vi "Solve2.vi"(8 "Error In":errorcluster, 11 "object in":refnum<class "2021_4.lvclass">) -> (0 "Error Out":errorcluster, 2 "Result":u64, 3 "object out":refnum<class "2021_4.lvclass">)   [LabVIEW 2020, in "2021_4.lvclass"]
uses:
  2021_4.lvclass
  2021_4.lvclass/2021_4.ctl
panel:
  out "LastBoard":i32
  out "Boards":bool[][][](array[boolean])
  out "Board":i32
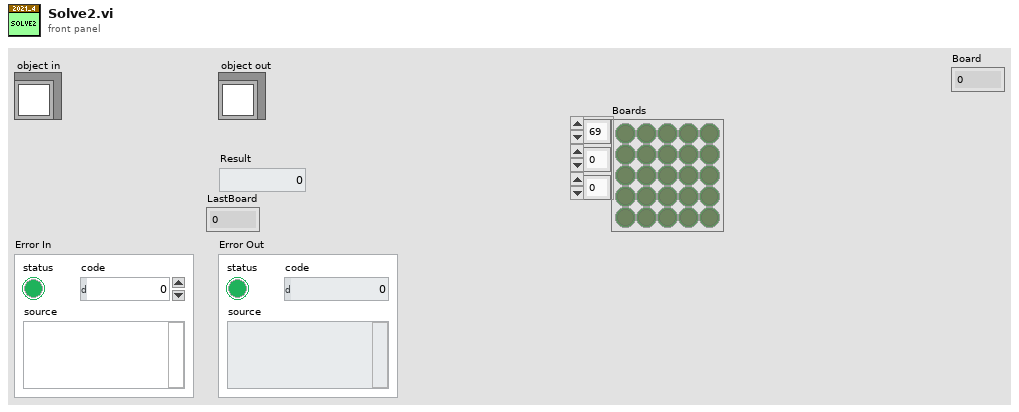
[diagram p1: front panel]
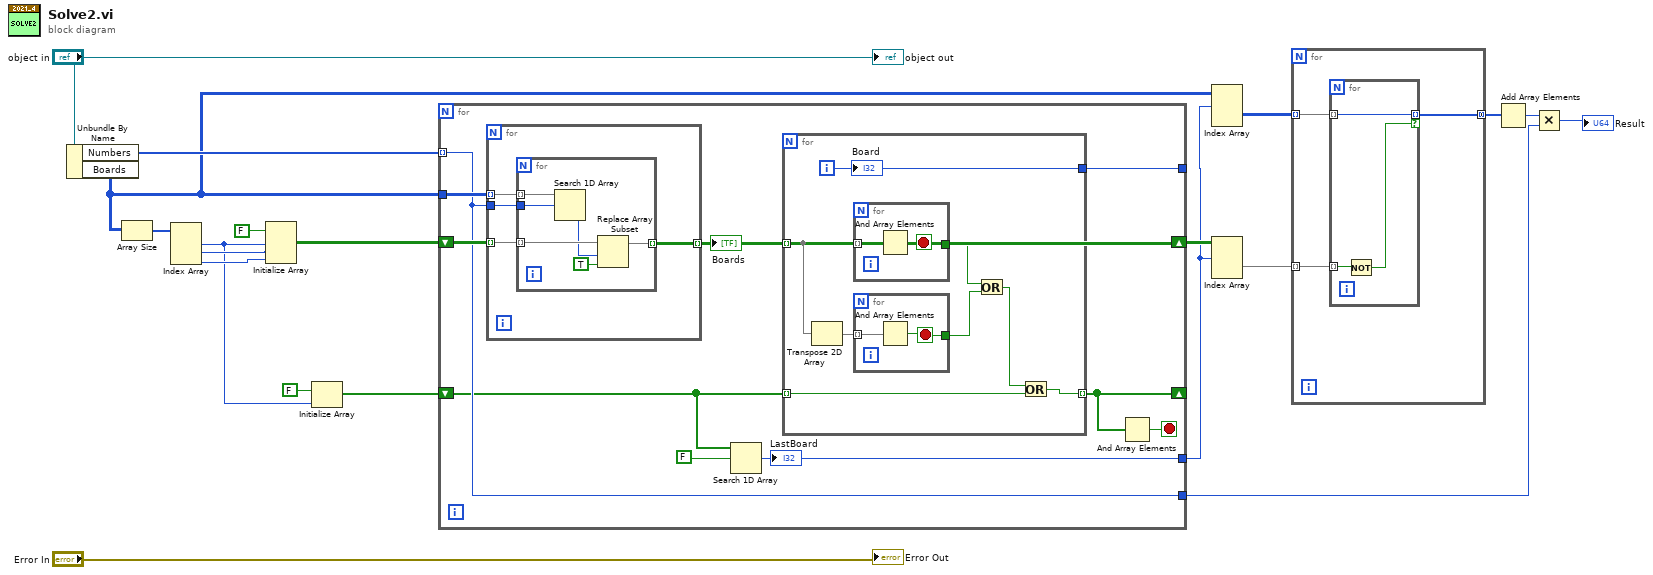
[diagram p0: block diagram]
diagram:
  n1 = Unbundle By Name("object in") -> ("Numbers"=w14:u32[], "Boards"=w12:i32[][][])
  n2 = Array Size(array=w12) -> (size(s)=w18:i32[])
  n3 = Index Array(array=w18) -> (element #1=w4:i32, element #2=w17:i32, element #3=w16:i32)  [unwired: 3 in]
  n4 = Initialize Array(FALSE, w4, w17, w16) -> (w13:bool[][][])
  n5 = Initialize Array(FALSE, w4) -> (w2:bool[])
  n6 = for {
    tunnel: w14 -> [w26] mode=indexing
    tunnel: w12 -> [w29]
    shift-right: [w28] -> w10
    shift-left: w13 -> [w30]
    tunnel: [w27] -> _
    tunnel: [w26] -> w6
    shift-right: [w25] -> _
    shift-left: w2 -> [w23]
    tunnel: [w21] -> w1
    stop <- w24 stop-if-true
    n7 = for {
      tunnel: w30 -> [w45] mode=indexing
      tunnel: w29 -> [w46] mode=indexing
      tunnel: w26 -> [w44]
      tunnel: [w43] -> w28 mode=indexing
      n8 = for {
        tunnel: w46 -> [w52] mode=indexing
        tunnel: w45 -> [w50] mode=indexing
        tunnel: w44 -> [w51]
        tunnel: [w47] -> w43 mode=indexing
        n9 = Search 1D Array(1D array=w52, element=w51) -> (index of element=w49:i32)  [unwired: 1 in]
        n10 = Replace Array Subset(array=w50, new element=TRUE ("new element/subarray"), index=w49) -> (w47:bool[])
      }
    }
    "Boards" <- w28
    n11 = Search 1D Array(1D array=w23, element=FALSE) -> (index of element=w21:i32)  [unwired: 1 in]
    "LastBoard" <- w21
    n12 = for {
      tunnel: w28 -> [w38] mode=indexing
      tunnel: [w34] -> w27
      tunnel: w23 -> [w33] mode=indexing
      tunnel: [w31] -> w25 mode=indexing
      i -> [w34]
      n13 = Transpose 2D Array(2D array=w38) -> (transposed array=w37:bool[][])
      n14 = for {
        tunnel: w38 -> [w42] mode=indexing
        tunnel: [w41] -> w36
        stop <- w41 stop-if-true
        n15 = And Array Elements(Boolean array=w42) -> (logical AND=w41:bool)
      }
      n16 = for {
        tunnel: w37 -> [w40] mode=indexing
        tunnel: [w39] -> w35
        stop <- w39 stop-if-true
        n17 = And Array Elements(Boolean array=w40) -> (logical AND=w39:bool)
      }
      n18 = Or(x=w36, y=w35) -> (x .or. y?=w32:bool)
      n19 = Or(x=w32, y=w33) -> (x .or. y?=w31:bool)
      "Board" <- w34
    }
    n20 = And Array Elements(Boolean array=w25) -> (logical AND=w24:bool)
  }
  n21 = Index Array(array=w12, index (dim 0)=w1) -> (element=w11:i32[][])  [unwired: 2 in]
  n22 = Index Array(array=w10, index (dim 0)=w1) -> (element=w9:bool[][])  [unwired: 2 in]
  n23 = for {
    tunnel: w11 -> [w55] mode=indexing
    tunnel: w9 -> [w54] mode=indexing
    tunnel: [w53] -> w8 mode=concatenating
    n24 = for {
      tunnel: w55 -> [w58] mode=indexing
      tunnel: w54 -> [w57] mode=indexing
      tunnel: [w58] -> w53 mode=indexing if=w56
      n25 = Not(x=w57) -> (.not. x?=w56:bool)
    }
  }
  n26 = Add Array Elements(numeric array=w8) -> (sum=w7:i32)
  n27 = Multiply(x=w7, y=w6) -> (x*y=→"Result":u32)
  "Error Out" <- "Error In"
  "object out" <- "object in"
